vi "pcfs_plot_data.vi"(8 "error in (no error)":errorcluster, 10 "data":dbl[](array[numeric]), 11 "scan_panel in":refnum<class "pcfs.lvclass">) -> (0 "error out":errorcluster, 3 "scan_panel out":refnum<class "pcfs.lvclass">)   [LabVIEW 2015, in "pcfs.lvclass"]
uses:
  pcfs.lvclass
  UI/panel_class/panel.lvclass/panel.ctl
  UI/panel_class/panel.lvclass
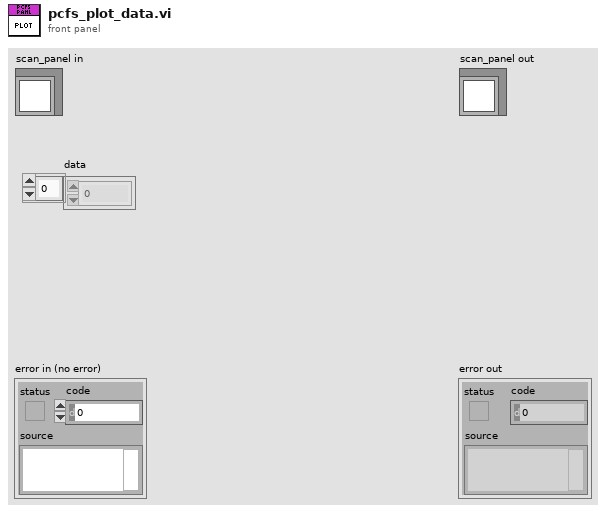
[diagram p1: front panel]
types:
  T1 = typedef "ui_user_events.ctl" = cluster{"update_xy_graph":refnum<user-event>, "update_graph":refnum<user-event>, "update_chart":refnum<user-event>, "update_map":refnum<user-event>, "event_loop_stop":refnum<user-event>, "keep_map":refnum<user-event>}
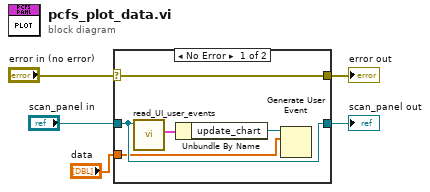
[diagram p0: block diagram]
diagram:
  n1 = case shown="No Error" "error in (no error)" {
    selector: "error in (no error)" -> [w10 w12]
    tunnel: [w10 w12] -> w4
    tunnel: [w9 w11] -> w2
    tunnel: "scan_panel in" -> [w9 w11]
    tunnel: "data" -> [w6 _]
    frame No Error {
      n2 = call "read_UI_user_events.vi"("panel in"=w9) -> ("ui_user_events"=w8:T1)  [unwired: 8 in, 2 out]
      n3 = Unbundle By Name(w8) -> ("update_chart"=w7:refnum<user-event>)
      n4 = Generate User Event(user event=w7, event data cluster=w6) -> ()  [unwired: 2 in, 2 out]
    }
    frame Error {
    }
  }
  "error out" <- w4
  "scan_panel out" <- w2
